vi "Add Folder.vi"(8 "error in (no error)":errorcluster, 11 "Server Creator Data in":T1) -> (0 "error out":errorcluster, 3 "Server Creator Data out":T1)   [LabVIEW 2025, in "Tools.lvlib"]
uses:
  Tools.lvlib
  Server Creator Data.ctl
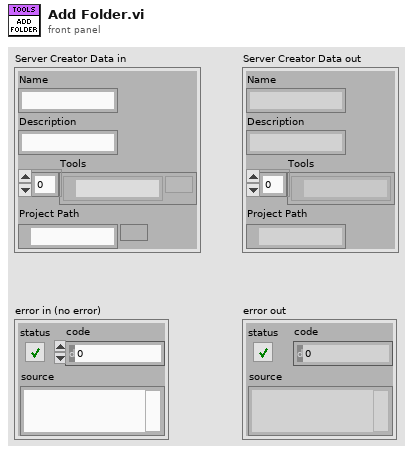
[diagram p1: front panel]
types:
  T1 = typedef "Tools.lvlib/Server Creator Data.ctl" = cluster{"Name":string, "Description":string, "Tools":path[], "Project Path":path}
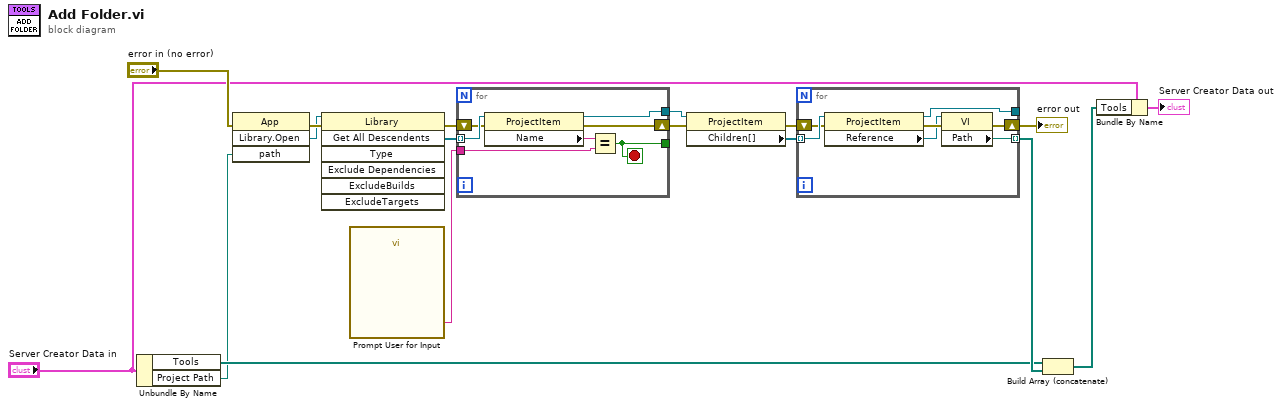
[diagram p0: block diagram]
diagram:
  n1 = Unbundle By Name("Server Creator Data in") -> ("Tools"=w13:path[], "Project Path"=w10:path)
  n2 = invoke class="App" method="Library.Open"(error in="error in (no error)", "path"=w10) -> (error out=w3:errorcluster, "Open Library"=w2:refnum<vi>)  [unwired: 2 in, 2 out]
  n3 = invoke class="Library" method="Get All Descendents"(reference=w2, error in=w3) -> (error out=w6:errorcluster, "All Descendents"=w7:refnum<vi>[])  [unwired: 5 in, 5 out]
  n4 = call "Prompt User for Input"() -> ("Folder Name"=w11:string)  [unwired: 17 in, 2 out]
  n5 = for {
    tunnel: w7 -> [w24] mode=indexing
    tunnel: [w23] -> w5
    shift-right: [w20] -> w4
    shift-left: w6 -> [w21]
    tunnel: [w19] -> _
    tunnel: w11 -> [w18]
    stop <- w19 stop-if-true
    n6 = property class="ProjectItem"(reference=w24, error in=w21) -> (reference out=w23:refnum<vi>, error out=w20:errorcluster, "Name"=w22:string)
    n7 = Equal?(x=w22, y=w18) -> (x = y?=w19:bool)
  }
  n8 = property class="ProjectItem"(reference=w5, error in=w4) -> (error out=w8:errorcluster, "Children[]"=w9:refnum<vi>[])  [unwired: 1 out]
  n9 = for {
    tunnel: w9 -> [w31] mode=indexing
    tunnel: [w30] -> _
    shift-right: [w27] -> w16
    shift-left: w8 -> [w29]
    tunnel: [w25] -> w15 mode=indexing
    n10 = property class="ProjectItem"(reference=w31, error in=w29) -> (reference out=w30:refnum<vi>, error out=w28:errorcluster, "Reference"=w26:refnum<vi>)
    n11 = property class="VI"(reference=w26, error in=w28) -> (error out=w27:errorcluster, "Path"=w25:path)  [unwired: 1 out]
  }
  "error out" <- w16
  n12 = Build Array (concatenate)(w13, w15) -> (w14:path[])
  n13 = Bundle By Name(cluster="Server Creator Data in", "Tools"=w14) -> (→"Server Creator Data out":T1)
